vi "run.archive.vi"(8 "error in":errorcluster, 11 "Client in":refnum<class "Client.lvclass">) -> (0 "error out":errorcluster, 3 "Client out":refnum<class "Client.lvclass">)   [LabVIEW 2020, in "Client.lvclass"]
doc: "Archives the run, hiding it from default views."
uses:
  Client.lvclass
  client.lvlib
panel:
  in  "rid":string
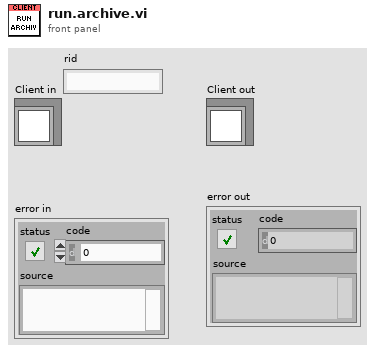
[diagram p1: front panel]
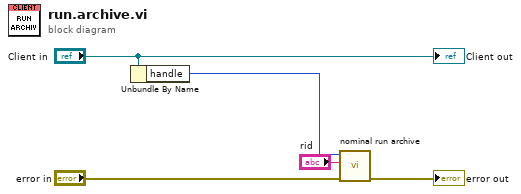
[diagram p0: block diagram]
diagram:
  n1 = Unbundle By Name("Client in") -> ("handle"=w3:i32)
  n2 = call "nominal run archive.vi"("error in (no error)"="error in", "rid"="rid", "client"=w3) -> ("error out"=→"error out":errorcluster)  [unwired: 7 in, 1 out]
  "Client out" <- "Client in"
